vi "ble_parse_scan_response.vi"(11 "Scan Response Data":u8[](array[numeric]) format="%02x") -> (3 "Array Scan Response":string[](array[string]))   [LabVIEW 2013]
uses:
  <vilib>/BLE/type_def/advertising_package_type.ctl
  Documents/desk/Kinvent/BLE112/BLE-Toolkit-LabVIEW-1.4.0.2/BLE-Toolkit-LabVIEW-1.4.0.2/ble_toolkit_source/type_def/address_type.ctl
panel:
  out "Friendly Name":string
  out "RSSI string":string
  out "Addvertiser Address Type":string
  in  "Address Type":T1 items=["Public", "Random"]
  out "MAC string OUT colon":string
  out "Advertising Package Type String":string
  in  "Advertising Package Type":T2 items=["Connectable Advertisement packet"=0, "Non Connectable Advertisement packet"=2, "Scan response packet"=4, "Discoverable advertisement packet"=6]
  out "RSSI (dBm)":i8
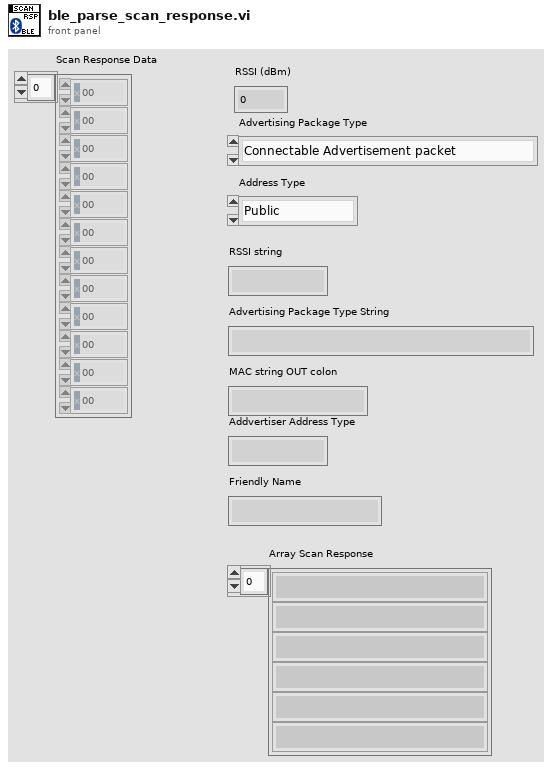
[diagram p1: front panel]
types:
  T1 = typedef "address_type.ctl" = u8
  T2 = typedef "advertising_package_type.ctl" = u8
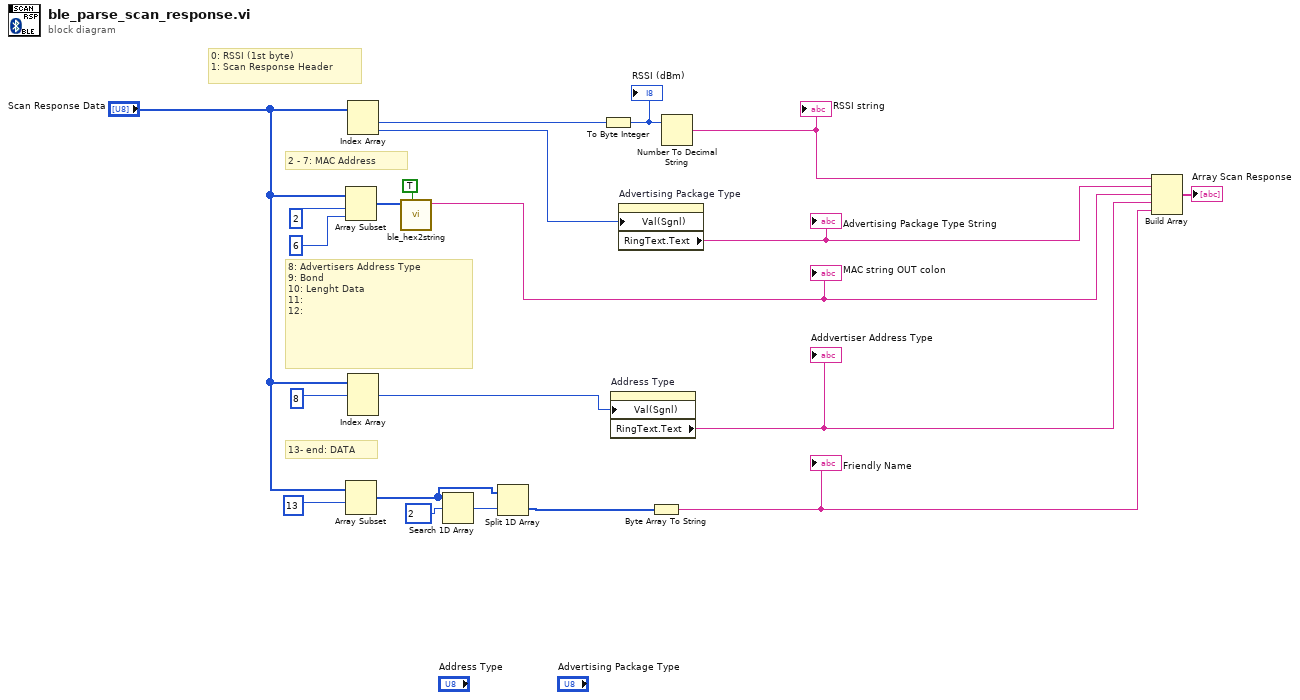
[diagram p0: block diagram]
diagram:
  # "13- end: DATA"
  # "8: Advertisers Address Type\n9: Bond\n10: Lenght Data\n11:\n12:"
  # "2 - 7: MAC Address"
  # "0: RSSI (1st byte)\n1: Scan Response Header"
  n1 = Array Subset(array="Scan Response Data", index=2, length=6) -> (w4:u8[])
  n2 = Array Subset(array="Scan Response Data", index=13 ("length")) -> (w7:u8[])  [unwired: 1 in]
  n3 = Index Array(array="Scan Response Data") -> (element #1=w21:u8, element #2=w14:u8)  [unwired: 2 in]
  n4 = Index Array(array="Scan Response Data", index #1=8 ("length")) -> (element #1=w13:u8)  [unwired: 2 in, 2 out]
  n5 = call <vilib>:"ble_hex2string.vi"("colon?(false)"=TRUE, "Byte Array IN (index0 LS byte)"=w4) -> ("HEX string OUT"=w3:string)  [unwired: 9 in]
  "MAC string OUT colon" <- w3
  n6 = Search 1D Array(1D array=w7, element=u8 2) -> (index of element=w8:i32)  [unwired: 1 in]
  n7 = Split 1D Array(array=w7, index=w8) -> (second subarray=w1:u8[])  [unwired: 1 out]
  n8 = To Byte Integer(number=w21) -> (8bit integer=w18:i8)
  "RSSI (dBm)" <- w18
  n9 = property on="Address Type" class="Ring (strict)"("Val(Sgnl)"=w13) -> ("RingText.Text"=w10:string)  [unwired: 2 in, 2 out]
  "Addvertiser Address Type" <- w10
  n10 = property on="Advertising Package Type" class="Ring (strict)"("Val(Sgnl)"=w14) -> ("RingText.Text"=w11:string)  [unwired: 2 in, 2 out]
  "Advertising Package Type String" <- w11
  n11 = Byte Array To String(unsigned byte array=w1) -> (string=w6:string)
  "Friendly Name" <- w6
  n12 = Number To Decimal String(number=w18) -> (decimal integer string=w12:string)  [unwired: 1 in]
  "RSSI string" <- w12
  n13 = Build Array(w12, w11, w3, w10, w6) -> (→"Array Scan Response":string[])
